vi "Arm.vi"(10 "Lift down":bool, 11 "Lift up":bool) -> ()   [LabVIEW 2014]
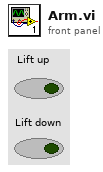
[diagram p1: front panel]
types:
  T1 = cluster{"Distance":dbl, "Rate":dbl, "Direction":bool, "Stopped":bool}
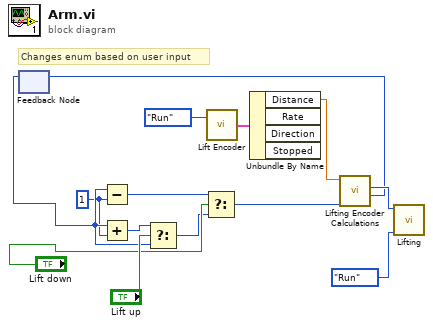
[diagram p0: block diagram]
diagram:
  w1 = 1
  # "Changes enum based on user input"
  n1 = feedback #1() -> (w5:i32)  [unwired: 1 in]
  n2 = Subtract(x=w5, y=w1) -> (x-y=w3:i32)
  n3 = Add(x=w5, y=w1) -> (x+y=w4:i32)
  n4 = Select(t=w4, s="Lift up", f=w5) -> (s? t:f=w2:i32)
  n5 = Select(t=w3, s="Lift down", f=w2) -> (s? t:f=w7:i32)
  n6 = call "Lift Encoder.vi"("Mode"=enum8{"Start", "Run", "Finish"}."Run") -> ("Lift Encoder"=w13:T1)  [unwired: 1 in]
  n7 = Unbundle By Name(w13) -> ("Distance"=w12:dbl)  [unwired: 3 out]
  n8 = call "Lifting Encoder Calculations.vi"("Position"=w7, "distance traveled"=w12) -> ("Current position"=w6:i32, "Direction"=w11:enum16{"stop", "up", "down"})  [unwired: 7 in]
  n9 = feedback-in #1(w6) -> ()
  n10 = call "Lifting.vi"("Direction"=w11, "Mode"=enum8{"Start", "Run", "Finish"}."Run") -> ()  [unwired: 4 in]
